vi "No Power User Choice.vi"(8 "error in (no error)":errorcluster, 10 "T button?":bool, 11 "PLC Data":T1) -> (0 "error out":errorcluster)   [LabVIEW 2016, in "PLC.lvlib"]
uses:
  PLC.lvlib
  Type definitions/PLC Data.ctl
  DAQ/TypeDefs/DAQ data.ctl
  DAQ/DAQ.lvlib
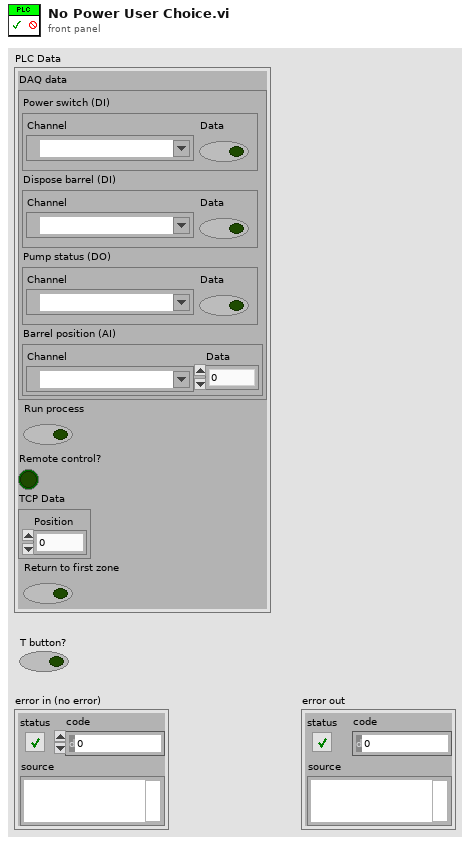
[diagram p1: front panel]
types:
  T1 = typedef "PLC.lvlib/PLC Data.ctl" = cluster{"DAQ data":T2, "Run process":bool, "Remote control?":bool, "TCP Data":cluster{"Position":dbl}, "Return to first zone":bool}
  T2 = typedef "DAQ.lvlib/DAQ data.ctl" = cluster{"Power switch (DI)":cluster{"Channel":tag, "Data":bool}, "Dispose barrel (DI)":cluster{"Channel":tag, "Data":bool}, "Pump status (DO)":cluster{"Channel":tag, "Data":bool}, "Barrel position (AI)":cluster{"Channel":tag, "Data":dbl}}
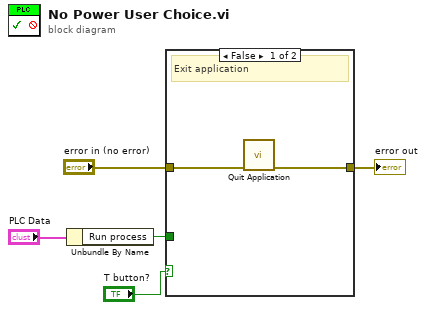
[diagram p0: block diagram]
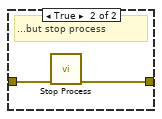
[diagram p3: hidden frame]
diagram:
  n1 = Unbundle By Name("PLC Data") -> ("Run process"=w4:bool)
  n2 = case shown="False" "T button?" {
    tunnel: "error in (no error)" -> [w7 w9]
    tunnel: [w6 w10] -> w3
    tunnel: w4 -> [_ w8]
    frame False {
      # "Exit application"
      n3 = call "Quit Application.vi"("error in"=w7) -> ("error out"=w6:errorcluster)  [unwired: 10 in]
    }
    frame True {
      # "Continue working..."
      n4 = case shown="False" w8 {
        tunnel: [w11 w12] -> w10
        tunnel: w9 -> [w11 w13]
        frame False {
          # "...and no change (idle)"
        }
        frame True {
          # "...but stop process"
          n5 = call "Stop Process.vi"("error in"=w13) -> ("error out"=w12:errorcluster)  [unwired: 10 in]
        }
      }
    }
  }
  "error out" <- w3
